vi "ConvertCmd2TlmArguments.vi"(4 "Input Command Arg":string[](array[string])) -> (1 "Output Telem Arg":string)   [LabVIEW 2010]
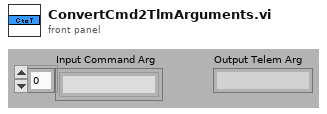
[diagram p1: front panel]
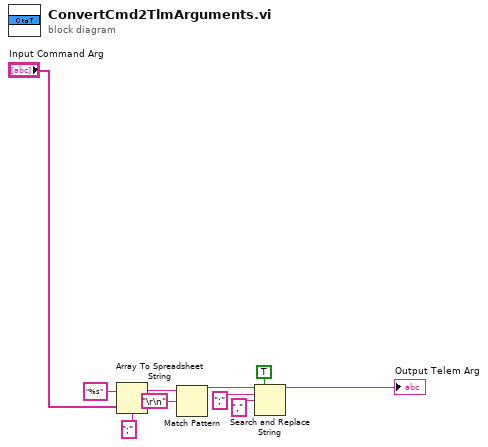
[diagram p0: block diagram]
diagram:
  n1 = Array To Spreadsheet String(delimiter (Tab)=";", array="Input Command Arg", 3:"%s" ("format string")) -> (spreadsheet string=w2:string)
  n2 = Match Pattern(string=w2, regular expression="\r\n") -> (before substring=w8:string)  [unwired: 4 out]
  n3 = Search and Replace String(replace all?=TRUE ("replace all? (F)"), input string=w8, search string=";", replace string="," ("replace string (\"\")")) -> (result string=→"Output Telem Arg":string)  [unwired: 4 in, 3 out]
